vi "Measure.vi"(8 "error in":errorcluster, 11 "Electronic Load in":refnum<class "Electronic Load.lvclass">) -> (0 "error out":errorcluster, 3 "Electronic Load out":refnum<class "Electronic Load.lvclass">)   [LabVIEW 2019, in "Electronic Load.lvlib" / "Electronic Load.lvclass"]
uses:
  Library/Electronic Load.lvclass
  C:/Users/Public/Documents/Development/builds/Instruments/Instruments.lvlibp/Library/Instruments.lvclass
  builds/Instruments/Instruments.lvlibp/Accessors/Read dt.vi
  builds/Instruments/Instruments.lvlibp/Library/Instruments.lvclass
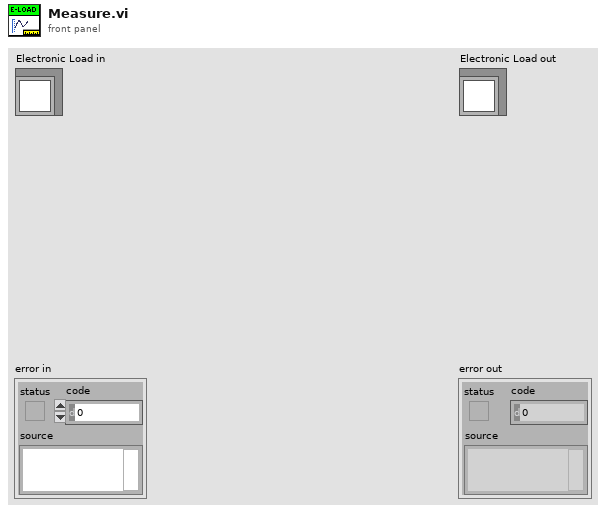
[diagram p1: front panel]
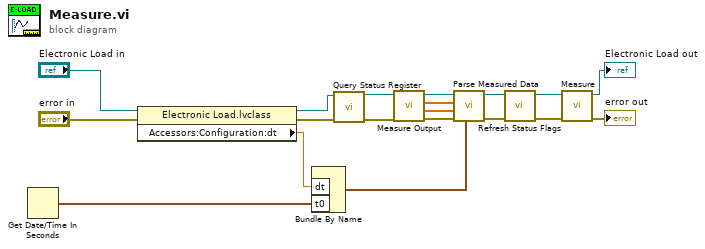
[diagram p0: block diagram]
diagram:
  n1 = Get Date/Time In Seconds() -> (seconds since 1Jan1904=w15:timestamp)
  n2 = property class="Electronic Load.lvclass"(reference="Electronic Load in", error in="error in") -> (reference out=w11:refnum<class "Electronic Load.lvclass">, error out=w13:errorcluster, "Accessors:Configuration:dt"=w10:dbl)
  n3 = Bundle By Name("dt"=w10, "t0"=w15) -> (w7:waveform(dbl))  [unwired: 1 in]
  n4 = call-dynamic "Query Status Register.vi"("error in (no error)"=w13, "Electronic Load in"=w11) -> ("error out"=w16:errorcluster, "Electronic Load out"=w17:refnum<class "Electronic Load.lvclass">)  [unwired: 8 in]
  n5 = call-dynamic "Measure Output.vi"("error in (no error)"=w16, "Electronic Load in"=w17) -> ("error out"=w8:errorcluster, "Current"=w6:dbl[], "Voltage"=w5:dbl[], "Electronic Load out"=w9:refnum<class "Electronic Load.lvclass">)  [unwired: 6 in]
  n6 = call "Parse Measured Data.vi"("Waveform Template"=w7, "error in"=w8, "Current"=w6, "Voltage"=w5, "Electronic Load in"=w9) -> ("error out"=w3:errorcluster, "Electronic Load out"=w4:refnum<class "Electronic Load.lvclass">)  [unwired: 5 in]
  n7 = call "Refresh Status Flags.vi"("error in"=w3, "Electronic Load in"=w4) -> ("error out"=w1:errorcluster, "Electronic Load out"=w2:refnum<class "Electronic Load.lvclass">)  [unwired: 8 in]
  n8 = call-parent "Measure.vi"("error in"=w1, "Instruments in"=w2) -> ("error out"=→"error out":errorcluster, "Instruments out"=→"Electronic Load out":refnum<class "Electronic Load.lvclass">)  [unwired: 8 in]
